vi "Move.vi"(8 "error in (no error)":errorcluster, 11 "Board_Game in":refnum<class "Board_Game.lvclass">) -> (0 "error out":errorcluster, 3 "Board_Game out":refnum<class "Board_Game.lvclass">)   [LabVIEW 2021, in "Board_Game.lvclass"]
uses:
  Board_Game.lvclass
  Board_Game.lvclass/Board_Game.ctl
  SnakeGame/Position.ctl
  SnakeGame/Snake.lvclass
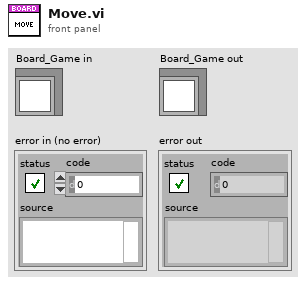
[diagram p1: front panel]
types:
  T1 = typedef "Direction.ctl" = enum16{"Up", "Down", "Left", "Right"}
  T2 = typedef "Position.ctl" = cluster{"X":u32, "Y":u32}
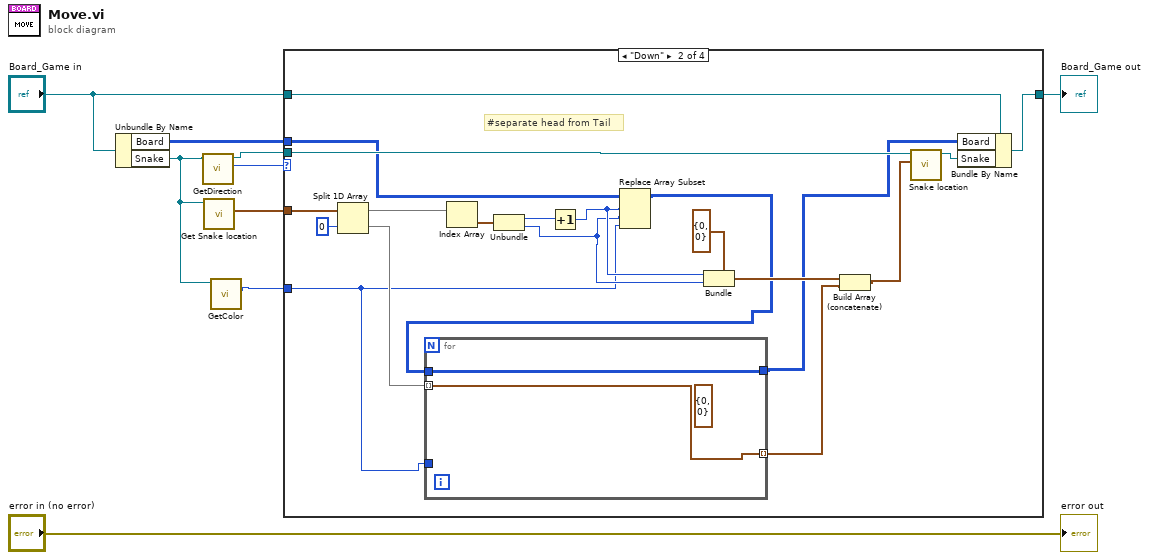
[diagram p0: block diagram]
diagram:
  n1 = Unbundle By Name("Board_Game in") -> ("Board"=w5:u32[][], "Snake"=w2:refnum<class "Snake.lvclass">)
  n2 = call-dynamic "GetDirection.vi"("Snake in"=w2) -> ("Direction"=w8:T1, "Snake out"=w4:refnum<class "Snake.lvclass">)  [unwired: 8 in, 1 out]
  n3 = call-dynamic "Get Snake location.vi"("Snake in"=w2) -> ("Snake location"=w6:T2[])  [unwired: 8 in, 2 out]
  n4 = call-dynamic "GetColor.vi"("SnakeGame in"=w2) -> ("Color"=w1:u32)  [unwired: 8 in, 2 out]
  n5 = case shown="\"Down\"" w8 {
    tunnel: "Board_Game in" -> [w10 w26 w33 w34]
    tunnel: [w10 w27 w33 w34] -> w7
    tunnel: w6 -> [_ w30 _ _]
    tunnel: w5 -> [_ w24 _ _]
    tunnel: w4 -> [_ w28 _ _]
    tunnel: w1 -> [_ w11 _ _]
    frame "Up", Default {
    }
    frame "Down" {
      # "#separate head from Tail"
      n6 = Split 1D Array(array=w30, index=0) -> (first subarray=w25:T2[], second subarray=w22:T2[])
      n7 = Index Array(array=w25) -> (element=w20:T2)  [unwired: 1 in]
      n8 = Unbundle(w20) -> ("X"=w19:u32, "Y"=w17:u32)
      n9 = Increment(x=w19) -> (x+1=w18:u32)
      n10 = Replace Array Subset(array=w24, new element=w11, index (row)=w18, index (col)=w17) -> (w13:u32[][])
      n11 = for {
        tunnel: w22 -> [w31] mode=indexing
        tunnel: w13 -> [w32]
        tunnel: [w32] -> w12
        tunnel: w11 -> [_]
        tunnel: [w31] -> w15 mode=indexing
        (unwired) T2 {"X"=0, "Y"=0} ("Position")
      }
      n12 = Bundle(cluster=T2 {"X"=0, "Y"=0} ("Position"), "X"=w18, "Y"=w17) -> (w16:T2)
      n13 = Build Array (concatenate)(w16, w15) -> (w14:T2[])
      n14 = call-dynamic "Snake location.vi"("Snake location"=w14, "Snake in"=w28) -> ("Snake out"=w23:refnum<class "Snake.lvclass">)  [unwired: 8 in, 1 out]
      n15 = Bundle By Name(cluster=w26, "Board"=w12, "Snake"=w23) -> (w27:refnum<class "Board_Game.lvclass">)
    }
    frame "Left" {
    }
    frame "Right" {
    }
  }
  "Board_Game out" <- w7
  "error out" <- "error in (no error)"
